vi "Get GObjs RectBound.vi"(8 "error in (no error)":errorcluster, 11 "GObjs":refnum<vi>[](array[refnum])) -> (0 "error out":errorcluster, 3 "Bound":T1)   [LabVIEW 2017]
doc: "Returns the bounding rectangle that encloses every front panel object in GObjs."
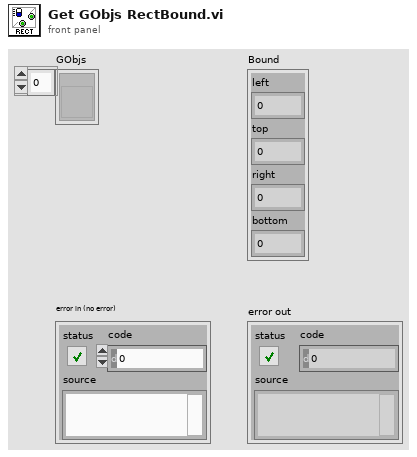
[diagram p1: front panel]
types:
  T1 = cluster{"left":i16, "top":i16, "right":i16, "bottom":i16}
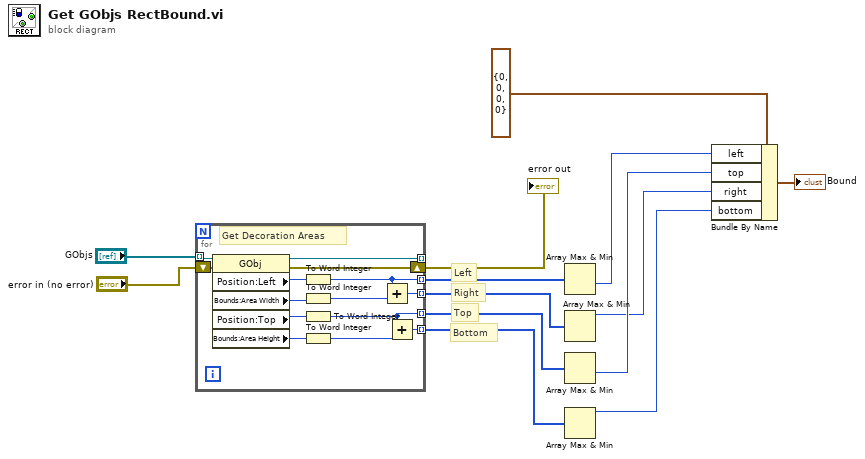
[diagram p0: block diagram]
diagram:
  # "Right"
  # "Left"
  # "Bottom"
  # "Top"
  n1 = for {
    tunnel: "GObjs" -> [w27] mode=indexing
    shift-right: [w25] -> w3
    shift-left: "error in (no error)" -> [w26]
    tunnel: [w24] -> _ mode=indexing
    tunnel: [w20] -> w13 mode=indexing
    tunnel: [w22] -> w12 mode=indexing
    tunnel: [w16] -> w11 mode=indexing
    tunnel: [w21] -> w10 mode=indexing
    # "Get Decoration Areas"
    n2 = property class="GObj"(reference=w27, error in=w26) -> (reference out=w24:refnum<vi>, error out=w25:errorcluster, "Position:Left"=w23:i32, "Bounds:Area Width"=w19:u32, "Position:Top"=w17:i32, "Bounds:Area Height"=w15:u32)
    n3 = To Word Integer(number=w23) -> (16bit integer=w20:i16)
    n4 = To Word Integer(number=w19) -> (16bit integer=w18:i16)
    n5 = To Word Integer(number=w17) -> (16bit integer=w16:i16)
    n6 = To Word Integer(number=w15) -> (16bit integer=w14:i16)
    n7 = Add(x=w20, y=w18) -> (x+y=w22:i16)
    n8 = Add(x=w16, y=w14) -> (x+y=w21:i16)
  }
  "error out" <- w3
  n9 = Array Max & Min(array=w13) -> (min value=w7:i16)  [unwired: 3 out]
  n10 = Array Max & Min(array=w12) -> (max value=w5:i16)  [unwired: 3 out]
  n11 = Array Max & Min(array=w11) -> (min value=w6:i16)  [unwired: 3 out]
  n12 = Array Max & Min(array=w10) -> (max value=w4:i16)  [unwired: 3 out]
  n13 = Bundle By Name(cluster=T1 {"left"=0, "top"=0, "right"=0, "bottom"=0} ("Snapped to bottom center"), "left"=w7, "top"=w6, "right"=w5, "bottom"=w4) -> (→"Bound":T1)
